vi "Close.vi"(8 "error in (no error)":errorcluster, 11 "Mouse Controller in":refnum<class "Mouse.lvclass">) -> (0 "error out":errorcluster)   [LabVIEW 2021, in "Mouse.lvclass"]
doc: "MIT Licence\nCopyright (c) 2024 David Grollier"
uses:
  Mouse.lvclass
  Mouse.lvclass/Mouse.ctl
  <vilib>/Utility/inputDevices.llb/closeMouse.vi
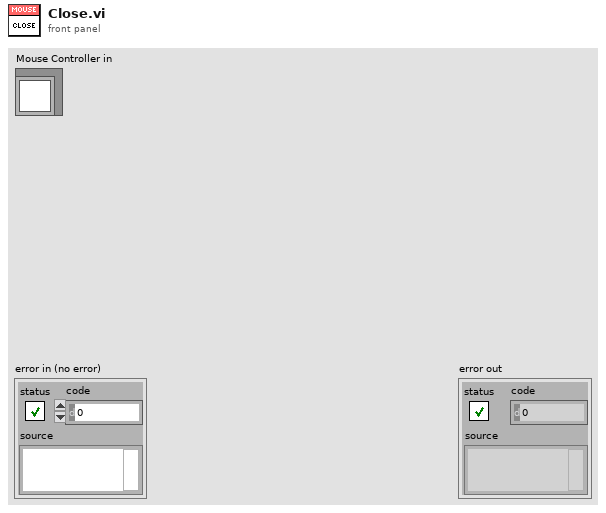
[diagram p1: front panel]
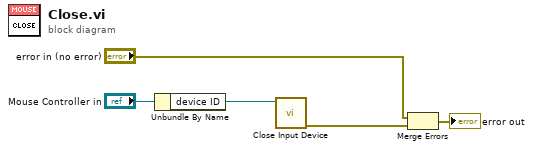
[diagram p0: block diagram]
diagram:
  n1 = Unbundle By Name("Mouse Controller in") -> ("device ID"=w1:refnum<k1>)
  n2 = call-poly <vilib>:"Close Input Device.vi"("device ID"=w1) -> ("error out"=w3:errorcluster)  [unwired: 9 in]
  n3 = Merge Errors("error in (no error)", w3) -> (→"error out":errorcluster)
